vi "Attenuator Print Test Panel.vi"(8 "error in (no error)":errorcluster, 11 "VI Reference":refnum<vi>) -> (0 "error out":errorcluster)   [LabVIEW 2011]
uses:
  <vilib>/Utility/miscctls.llb/LVPrintingMarginsTypeDef.ctl
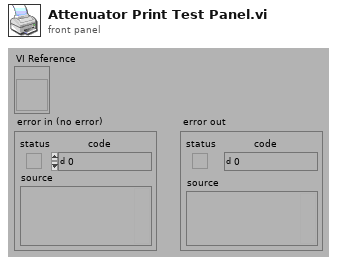
[diagram p1: front panel]
types:
  T1 = enum32{"Portrait", "Landscape", "Rotated Portrait", "Rotated Landscape"}
  T2 = typedef "LVPrintingMarginsTypeDef.ctl" = cluster{"Top":sgl, "Left":sgl, "Bottom":sgl, "Right":sgl, "Measurement System":enum8{"Inches", "cm"}}
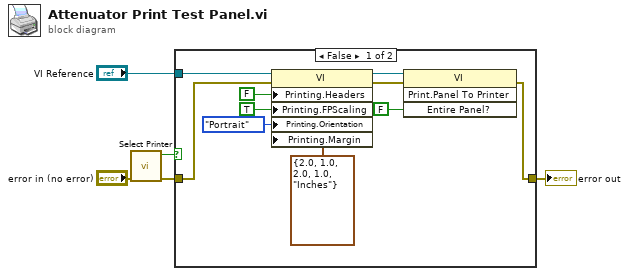
[diagram p0: block diagram]
diagram:
  n1 = call "Select Printer.vi"("error in (no error)"="error in (no error)") -> ("error out"=w2:errorcluster, "Canceled?"=w1:bool)  [unwired: 9 out]
  n2 = case shown="False" w1 {
    tunnel: "VI Reference" -> [w15 _]
    tunnel: [w14 w16] -> w4
    tunnel: w2 -> [w13 w16]
    frame False {
      n3 = property class="VI"(reference=w15, error in=w13, "Printing.Headers"=FALSE ("Printing:Page Headers?"), "Printing.FPScaling"=TRUE ("Printing:Front Panel Scaling?"), "Printing.Orientation"=T1."Portrait" ("Printing:Page Orientation"), "Printing.Margin"=T2 {"Top"=2.0, "Left"=1.0, "Bottom"=2.0, "Right"=1.0, "Measurement System"=enum."Inches"} ("Printing:Margins")) -> (reference out=w10:refnum<vi>, error out=w11:errorcluster)
      n4 = invoke class="VI" method="Print.Panel To Printer"(reference=w10, error in=w11, "Entire Panel?"=FALSE) -> (error out=w14:errorcluster)  [unwired: 1 in, 3 out]
    }
    frame True {
    }
  }
  "error out" <- w4
